vi "GUI_TREX.vi"(8 "error IO":errorcluster) -> (0 "error IO 2":errorcluster)   [LabVIEW 2013]
uses:
  shared programs/GUI_Template/GUI_master/tcp_new_data_event.ctl
  shared programs/GUI_Template/GUI_master/tcp new data cluster.ctl
  VIremote/VIremote.llb/VIremoteFunction.ctl
panel:
  in  "delay.Channel_A::2":dbl=0.001 caption="Lamp Delay" format="%_12f"
  in  "delay.Channel_D::2":dbl=0.001 caption="Q Switch Delay" format="%_12f"
  in  "stepsize::1":dbl=0.001 caption="Step Size" format="%^_5e"
  in  "relativeMove.Axis 3pos::1":bool
  in  "relativeMove.Axis 3neg::1":bool caption="Up Button"
  in  "relativeMove.Axis 2pos::1":bool
  in  "relativeMove.Axis 2neg::1":bool caption="Up Button"
  in  "relativeMove.Axis 1pos::1":bool
  in  "relativeMove.Axis 1neg::1":bool caption="Up Button"
  in  "Position.Axis 3::1":dbl=0.001 caption="OAP vertical" format="%^_5e"
  in  "Position.Axis 2::1":dbl=0.001 caption="OAP horizontal (mm)" format="%^_5e"
  in  "Position.Axis 1::1":dbl=0.001 caption="comp4" format="%^_5e"
  in  "GUIdevice 2":string="TREX-Preamp2Delay"
  out "hor?":dbl=0.001 caption="OAP vertical" format="%_4p"
  out "vert?":dbl=0.001 caption="OAP horizontal" format="%_4p"
  out "comp4":dbl=0.001 format="%_4p"
  out "tcp data event":T1
  in  "GUIdevice 1":string="TREX_ESP_300_1"
  in  "insert tag":bool=TRUE
  in  "stop":bool
  # "TREX CONTROL CENTER"
  # "Preamp 2"
  # "in meters..."
  # "OAP and Compressor"
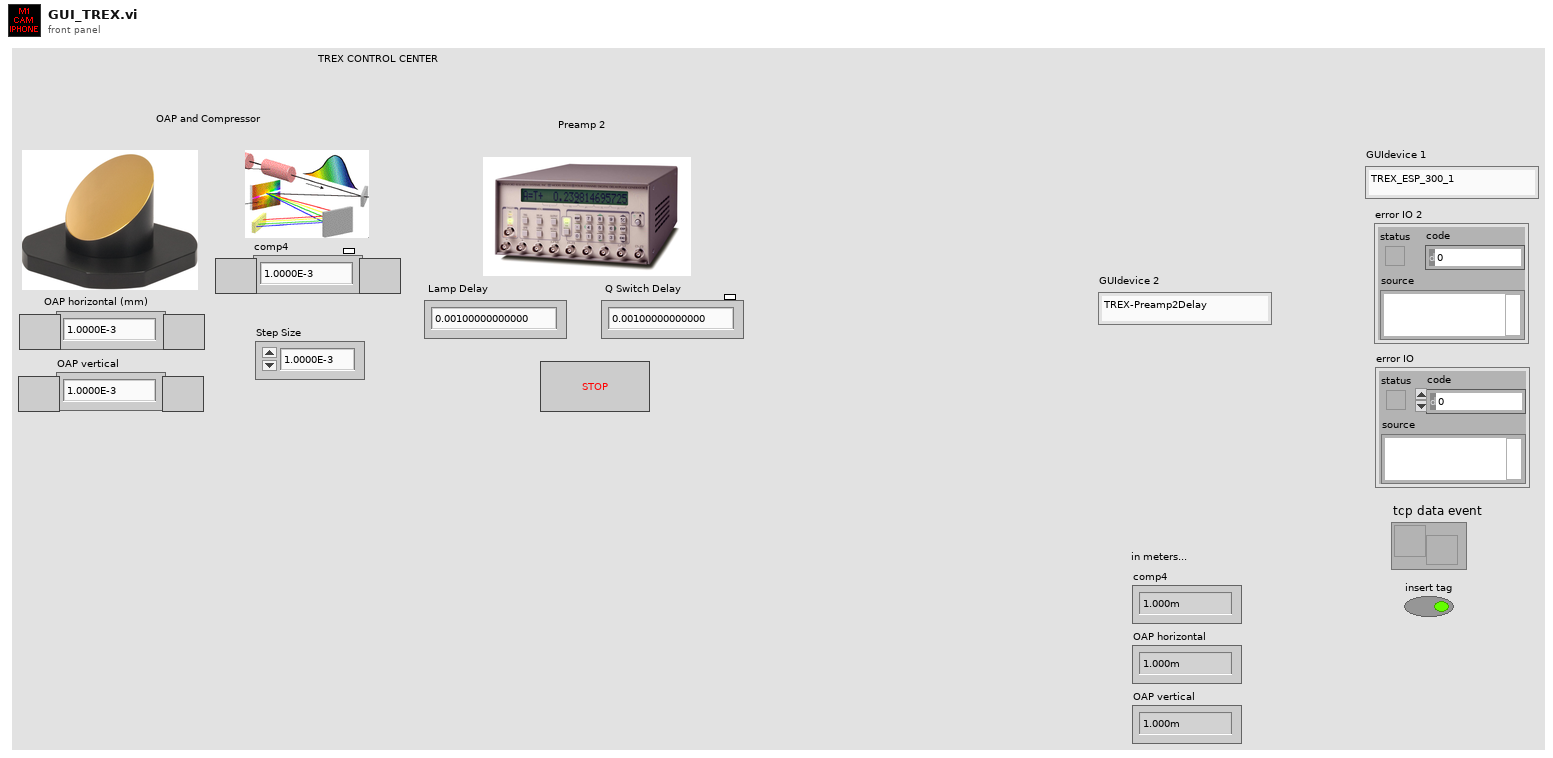
[diagram p1: front panel]
types:
  T1 = typedef "tcp_new_data_event.ctl" = refnum<user-event>
  T2 = typedef "tcp new data cluster.ctl" = cluster{"EventEnum":enum16{"new data", "connection status update"}, "Device name":string}
  T3 = typedef "VIremoteFunction.ctl" = enum16{"Do nothing", "Stop controller", "Close this connection", "Show info panel", "Set VI to control", "Set Accelerometer freq (Hz)", "Show Alert message", "Start Sound Input", "Stop Sound Input", "Set Volume (0-100)", "Set sound output Speaker", "Set sound output Receiver", "Play Sound", "Repeat Sound", "Stop Sound", "Pause Sound", "Resume Sound", "Set panel width of caller (320 or 480)", "Set Panel Size to Portrait", "Set Panel Size to Landscape", "Set Panel Size as Current Orientation", "Allow all UI Orientations", "Send user notification", "Disable Scrolling", "Normal Scrolling", "Page Scrolling", "Set Scroll Offset", "Page Indicator Position"}
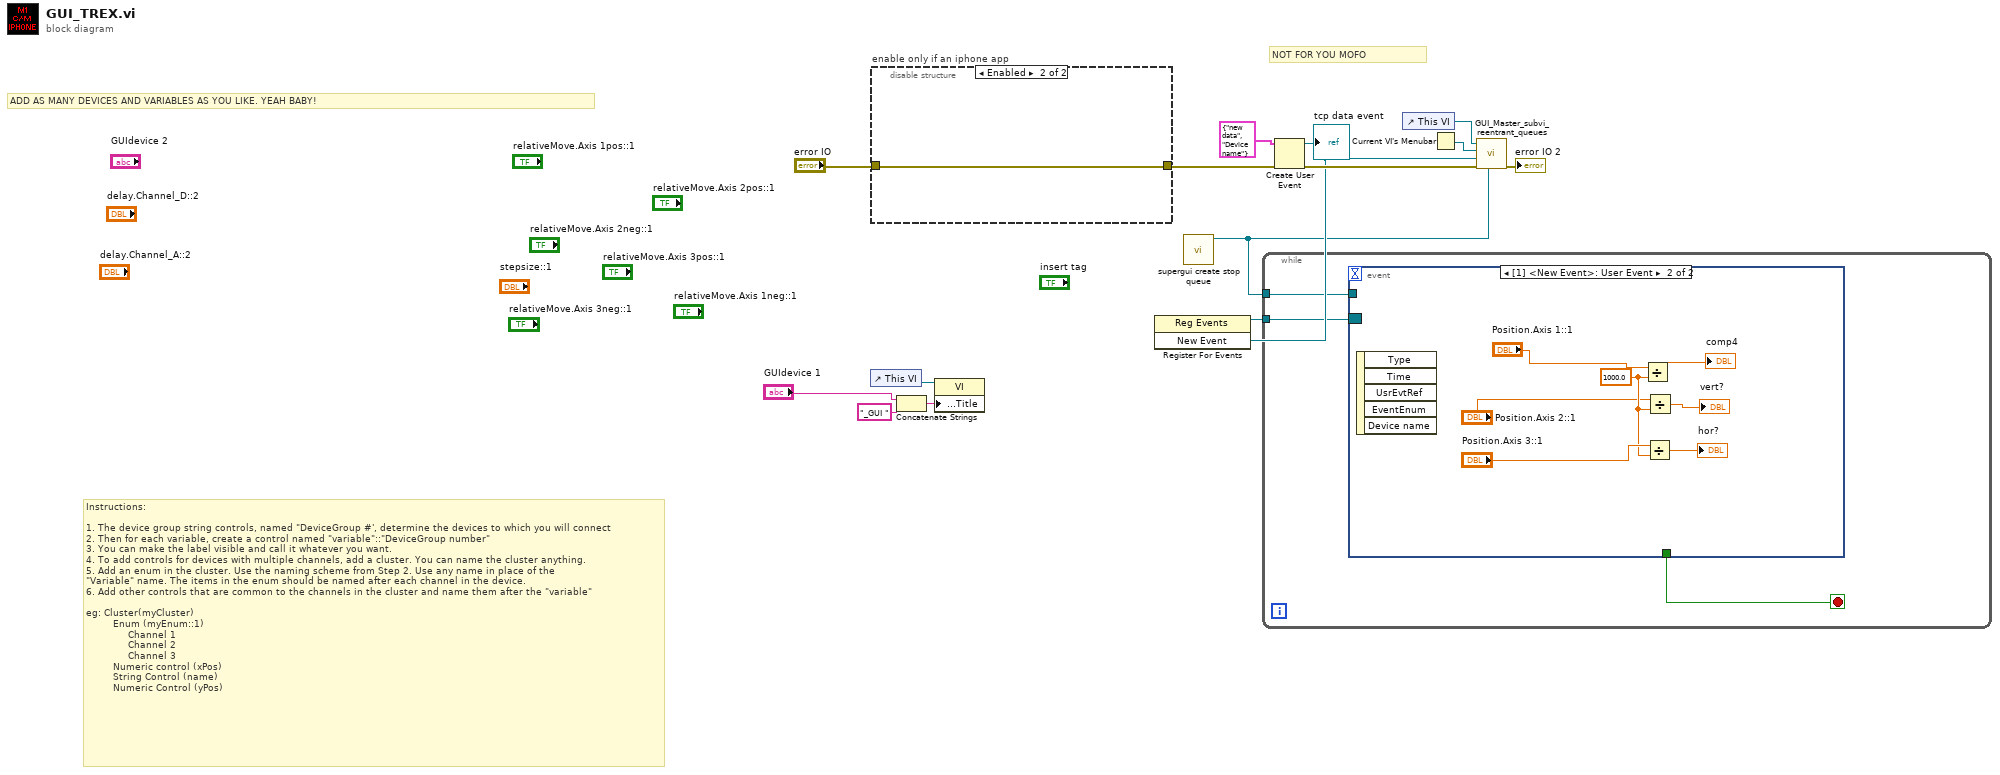
[diagram p0: block diagram]
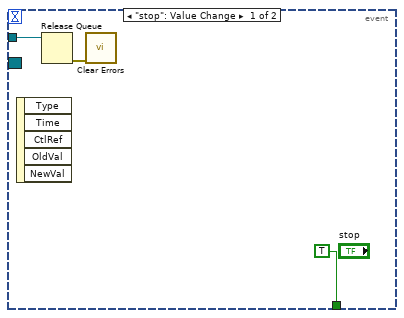
[diagram p2: hidden frame]
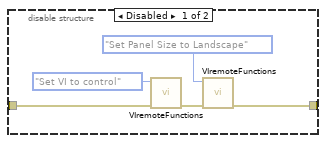
[diagram p3: hidden frame]
diagram:
  # "NOT FOR YOU MOFO"
  # "Instructions:\n\n1. The device group string controls, named \"DeviceGroup #', determine the devices to which you will connect\n2. Then for each variable, create a control named \"variable\"::\"DeviceGroup number\"\n3. You can make the label visible and call it whatever you want.\n4. To add controls for devices with multiple channels, add a cluster. You can name the cluster anything.\n5. Add an enum in the cluster. Use the naming scheme from Step 2. Use any name in place of the \n\"Variable\" name. The items in the enum should be named after each channel in the device. \n6. Add other controls that are common to the channels in the cluster and name them after the \"variable\"\n\neg: Cluster(myCluster)\n         Enum (myEnum::1)\n              Channel 1 \n              Channel 2\n              Channel 3\n         Numeric control (xPos)\n         String Control (name)\n         Numeric Control (yPos)"
  # "ADD AS MANY DEVICES AND VARIABLES AS YOU LIKE. YEAH BABY!"
  n1 = control-ref of="This VI"() -> (w4:refnum<vi>)
  n2 = disable-structure "enable only if an iphone app" shown="Enabled" {
    disable-tunnel: [w16 w20] -> w9
    disable-tunnel: "error IO" -> [w15 w20]
    frame Disabled {
      n3 = call "VIremoteFunctions.vi"("error in (no error)"=w15, "Function"=VIremoteFunction."Set VI to control") -> ("error out"=w17:errorcluster)  [unwired: 4 in, 5 out]
      n4 = call "VIremoteFunctions.vi"("error in (no error)"=w17, "Function"=VIremoteFunction."Set Panel Size to Landscape") -> ("error out"=w16:errorcluster)  [unwired: 4 in, 5 out]
    }
    frame Enabled {
    }
  }
  n5 = Concatenate Strings("GUIdevice 1", "_GUI ") -> (w3:string)
  n6 = property class="VI"(reference=w4, "Front Panel.Title"=w3) -> ()  [unwired: 1 in, 2 out]
  n7 = call "supergui create stop queue.vi"() -> ("STOP Queue out"=w5:refnum<queue>)  [unwired: 11 in]
  n8 = Create User Event(user event datatype=T2 {"EventEnum"=enum."new data", "Device name"="Device name"} ("New Event"), error in=w9) -> (user event=w7:refnum<user-event>, error out=w10:errorcluster)
  "tcp data event" <- w7
  n9 = register-events(w7) -> (reference out=w6:refnum<event-registration>)  [unwired: 2 in, 1 out]
  n10 = while {
    tunnel: w6 -> [w22]
    tunnel: w5 -> [w21]
    stop <- w23 stop-if-true
    n11 = event shown="[1] <New Event>: User Event" {
      selector: w22 -> [_ _]
      dyn-events: _ -> [_ _]
      timeout: _ -> [_ _]
      tunnel: [TRUE ("stop") _] -> w23
      tunnel: w21 -> [w24 _]
      event "stop": Value Change {
        n12 = event-data() -> ()  [unwired: 1 in, 5 out]
        n13 = Release Queue(queue=w24) -> (error out=w25:errorcluster)  [unwired: 2 in, 2 out]
        n14 = call <vilib>:"Clear Errors.vi"("error in (no error)"=w25) -> ()  [unwired: 6 in, 1 out]
      }
      event User Event {
        w32 = 1000.0 ("y")
        n15 = event-data() -> ()  [unwired: 1 in, 5 out]
        n16 = Divide(x="Position.Axis 1::1", y=w32) -> (x/y=→"comp4":dbl)
        n17 = Divide(x="Position.Axis 3::1", y=w32) -> (x/y=→"hor?":dbl)
        n18 = Divide(x="Position.Axis 2::1", y=w32) -> (x/y=→"vert?":dbl)
      }
    }
  }
  n19 = control-ref of="This VI"() -> (w13:refnum<vi>)
  n20 = Current VI's Menubar() -> (w12:refnum<k9>)
  n21 = call "GUI_Master_subvi_reentrant_queues.vi"("STOP Queue in"=w5, "error in (no error)"=w10, "tcp data event"=w7, "Caller menu reference"=w12, "Caller VI ref"=w13) -> ("error out"=→"error IO 2":errorcluster)  [unwired: 6 in]
